vi "produitProcess_GFV_etatSuivant.vi"(8 "etatNormal":T1, 9 "etatPrioritaire":T1=enum."safe", 10 "prioritaire?":bool=TRUE, 11 "fonction":T2) -> (1 "prioritaire? out":bool, 3 "etatSuivant":T1)   [LabVIEW 2020]
uses:
  Modules/Fonction Standard/Bouton & Control/setget.ctl
  enum_etatsMarche.ctl
  Modules/FS/60_FS_Controles/60_FS_SetGet.ctl
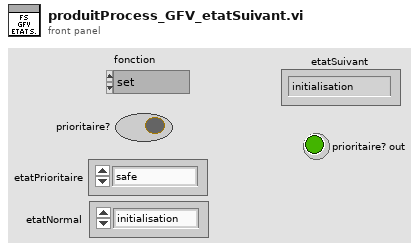
[diagram p1: front panel]
types:
  T1 = typedef "enum_etatsMarche.ctl" = enum16{"initialisation", "safe", "armement", "production", "maintenance", "quitter"}
  T2 = typedef "setget.ctl" = enum16{"set", "get"}
  T3 = typedef "60_FS_SetGet.ctl" = enum16{"set", "get"}
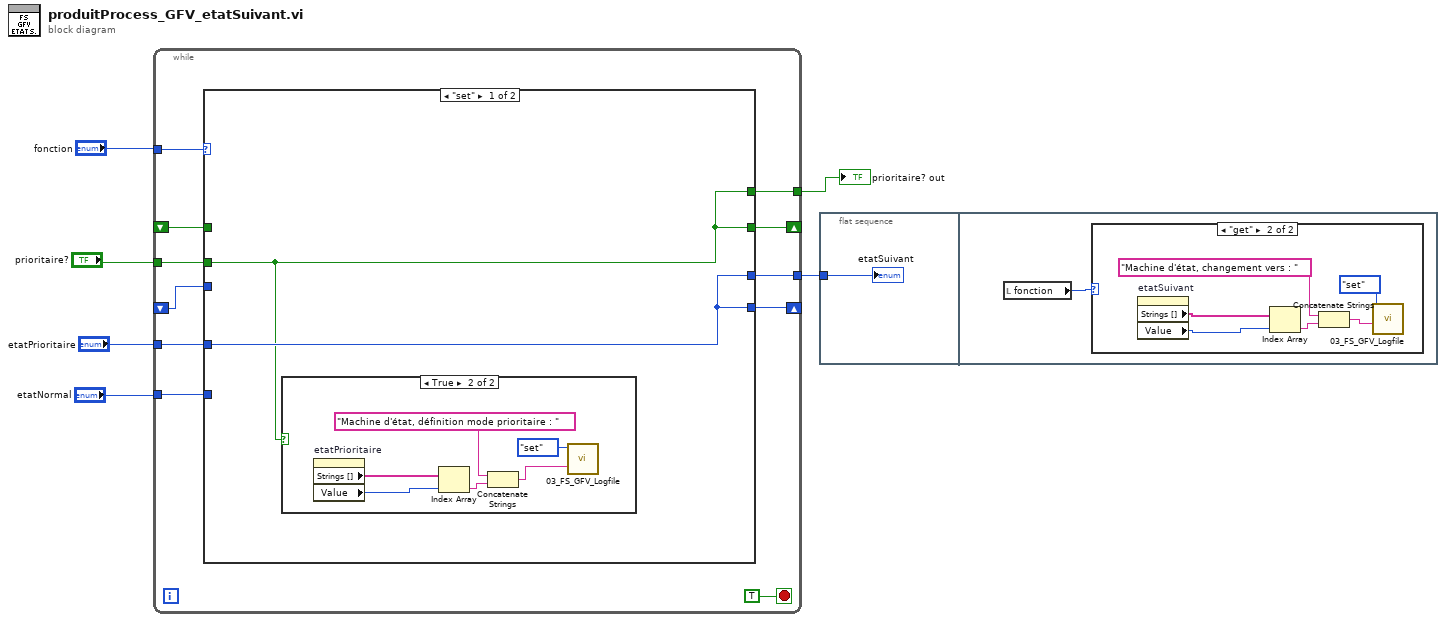
[diagram p0: block diagram]
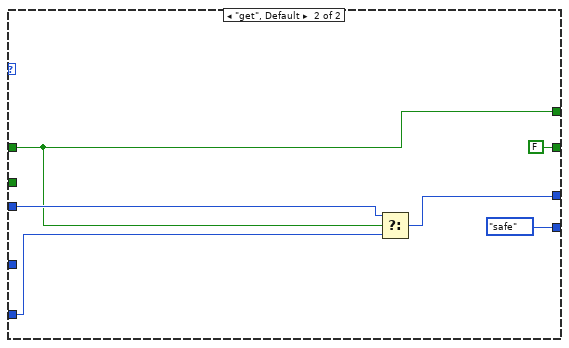
[diagram p4: hidden frame]
diagram:
  n1 = while {
    tunnel: "fonction" -> [w16]
    shift-right: [w15] -> _
    shift-left: _ -> [w13]
    tunnel: "prioritaire?" -> [w14]
    tunnel: "etatPrioritaire" -> [w12]
    shift-right: [w11] -> _
    shift-left: _ -> [w10]
    tunnel: "etatNormal" -> [w9]
    tunnel: [w8] -> w4
    tunnel: [w7] -> w3
    stop <- TRUE stop-if-true
    n2 = case shown="\"set\"" w16 {
      tunnel: [w18 FALSE ("prioritaire?")] -> w15
      tunnel: w14 -> [w18 _]
      tunnel: w13 -> [_ w30]
      tunnel: w12 -> [w19 _]
      tunnel: [w19 enum_etatsMarche."safe" ("etatPrioritaire")] -> w11
      tunnel: w10 -> [_ w31]
      tunnel: w9 -> [_ w27]
      tunnel: [w18 w30] -> w8
      tunnel: [w19 w29] -> w7
      frame "set" {
        n3 = case shown="True" w18 {
          frame False {
          }
          frame True {
            n4 = property on="etatPrioritaire" class="Enum (strict)"() -> ("Strings []"=w21:string[], "Value"=w20:T1)  [unwired: 2 in, 2 out]
            n5 = Index Array(array=w21, index=w20) -> (element=w23:string)
            n6 = Concatenate Strings("Machine d'état, définition mode prioritaire : " ("chaîne"), w23) -> (w22:string)
            n7 = call "03_FS_GFV_Logfile.vi"("Chaîne"=w22, "States"=60_FS_SetGet."set") -> ()  [unwired: 8 in, 2 out]
          }
        }
      }
      frame "get", Default {
        n8 = Select(t=w31, s=w30, f=w27) -> (s? t:f=w29:T1)
      }
    }
  }
  "prioritaire? out" <- w4
  n9 = flat-sequence {
    tunnel: w3 -> [w32]
    frame #0 {
      "etatSuivant" <- w32
    }
    frame #1 {
      n10 = local read "fonction"() -> (w33:T2)
      n11 = case shown="\"get\"" w33 {
        frame "set", Default {
        }
        frame "get" {
          n12 = property on="etatSuivant" class="Enum (strict)"() -> ("Strings []"=w34:string[], "Value"=w35:T1)  [unwired: 2 in, 2 out]
          n13 = Index Array(array=w34, index=w35) -> (element=w37:string)
          n14 = Concatenate Strings("Machine d'état, changement vers : " ("chaîne"), w37) -> (w39:string)
          n15 = call "03_FS_GFV_Logfile.vi"("Chaîne"=w39, "States"=60_FS_SetGet."set") -> ()  [unwired: 8 in, 2 out]
        }
      }
    }
  }
